vi "Teleop.vi"(10 "Match Info":T1={"Autonomous Elapsed Seconds"=0.0, "TeleOp Elapsed Seconds"=0.0, "Disabled Elapsed Seconds"=0.0, "Visited Autonomous"=FALSE, "Visited TeleOp"=FALSE, "Visited Disabled"=FALSE, "Autonomous Settings"={"Autonomous Style"=enum."Independent", "VI Refnum"=refnum}}, 11 "Call Context":T2) -> ()   [LabVIEW 2014]
doc: "This VI is called for each TeleOp packet received from the DS where the robot is not disabled. It is often used to read from the joysticks and update I/O or to update setpoints for timed control loops. It should complete and return within 20 milliseconds or it may miss DS packets."
uses:
  <vilib>/Rock Robotics/WPI/DriverStation/WPI_DriverStationDerivedRobotMode.ctl
  <vilib>/Rock Robotics/WPI/DriverStation/WPI_DriverStationMatch Info.ctl
  <vilib>/Rock Robotics/WPI/Joystick/WPI_JoystickGetSetRefNum.vi
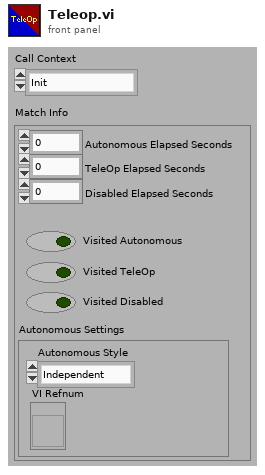
[diagram p1: front panel]
types:
  T1 = typedef "WPI_DriverStationMatch Info.ctl" = cluster{"Autonomous Elapsed Seconds":dbl, "TeleOp Elapsed Seconds":dbl, "Disabled Elapsed Seconds":dbl, "Visited Autonomous":bool, "Visited TeleOp":bool, "Visited Disabled":bool, "Autonomous Settings":cluster{"Autonomous Style":enum16{"Iterative", "Independent"}, "VI Refnum":refnum<vi>}}
  T2 = typedef "WPI_DriverStationDerivedRobotMode.ctl" = enum16{"Init", "Execute", "Stop"}
  T3 = typedef "WPI_SolenoidDevRef.ctl" = cluster{"DevStatus":errorcluster, "Pneumatics Control Module":u8, "Forward Solenoid Channel":T4, "Reverse Solenoid Channel":T4}
  T4 = typedef "WPI_SolenoidChannel.ctl" = enum8{"Solenoid 0", "Solenoid 1", "Solenoid 2", "Solenoid 3", "Solenoid 4", "Solenoid 5", "Solenoid 6", "Solenoid 7", "Invalid"}
  T5 = typedef "WPI_JoystickDevRef.ctl" = cluster{"Device":T6}
  T6 = typedef "WPI_JoystickDeviceEnum.ctl" = enum16{"USB 0", "USB 1", "USB 2", "USB 3", "USB 4", "USB 5"}
  T7 = typedef "WPI_DigitalInputDevRef.ctl" = cluster{"DevStatus":errorcluster, "DIO Channel":T8, "Controller":T9}
  T8 = typedef "FPGA_DIOChannel.ctl" = enum8{"DIO 0", "DIO 1", "DIO 2", "DIO 3", "DIO 4", "DIO 5", "DIO 6", "DIO 7", "DIO 8", "DIO 9", "DIO MXP 0", "DIO MXP 1", "DIO MXP 2", "DIO MXP 3", "DIO MXP 4", "DIO MXP 5", "DIO MXP 6", "DIO MXP 7", "DIO MXP 8", "DIO MXP 9", "DIO MXP 10", "DIO MXP 11", "DIO MXP 12", "DIO MXP 13", "DIO MXP 14", "DIO MXP 15", "Invalid"}
  T9 = typedef "FPGA_TypedefDigitalModule.ctl" = enum16{"Controller 1"}
  T10 = typedef "WPI_AnalogChannelDevRef.ctl" = cluster{"DevStatus":errorcluster, "Controller":T11, "Analog Channel":T12}
  T11 = typedef "FPGA_TypedefAnalogModule.ctl" = enum16{"Controller 1"}
  T12 = typedef "FPGA_AIChannel.ctl" = enum8{"AI 0", "AI 1", "AI 2", "AI 3", "AI MXP 0", "AI MXP 1", "AI MXP 2", "AI MXP 3", "Invalid"}
  T13 = typedef "WPI_MotorControlDeviceRef.ctl" = cluster{"DeviceStatus":errorcluster, "Type":T14, "PWM":cluster{"Controller":T9, "PWM Channel":T15, "DeadBand":T16}, "CAN":cluster{"Device Number":u8, "Control Mode":T17, "Semaphore":T18, "Max Vout":dbl, "TalonSRX Control Mode":T19}, "Invert":bool, "TransformRef":T20, "InvTransformRef":T20}
  T14 = typedef "WPI_MotorControlType.ctl" = enum16{"PWM", "CAN", "CANTalonSRX"}
  T15 = typedef "FPGA_DIOPWMChannel.ctl" = enum8{"PWM 0", "PWM 1", "PWM 2", "PWM 3", "PWM 4", "PWM 5", "PWM 6", "PWM 7", "PWM 8", "PWM 9", "PWM MXP 0", "PWM MXP 1", "PWM MXP 2", "PWM MXP 3", "PWM MXP 4", "PWM MXP 5", "PWM MXP 6", "PWM MXP 7", "PWM MXP 8", "PWM MXP 9", "Invalid"}
  T16 = typedef "WPI_PWMDeadband.ctl" = cluster{"Name":string, "maxPositivePwm":i32, "minPositivePwm":i32, "centerPwm":i32, "maxNegativePwm":i32, "minNegativePwm":i32, "angularRange":u16}
  T17 = typedef "WPI_CANJaguar_ControlMode.ctl" = enum8{"Percent VBus", "Current", "Speed", "Position", "Voltage"}
  T18 = typedef "Semaphore RefNum" = refnum<k1>
  T19 = typedef "WPI_CANTalonSRX_APIControlMode.ctl" = enum8{"Percent VBus", "Speed", "Position", "Slave", "Unchanged / Invalid"}
  T20 = typedef "WPI_PWMTransform_ConPane.ctl" = refnum<vi>
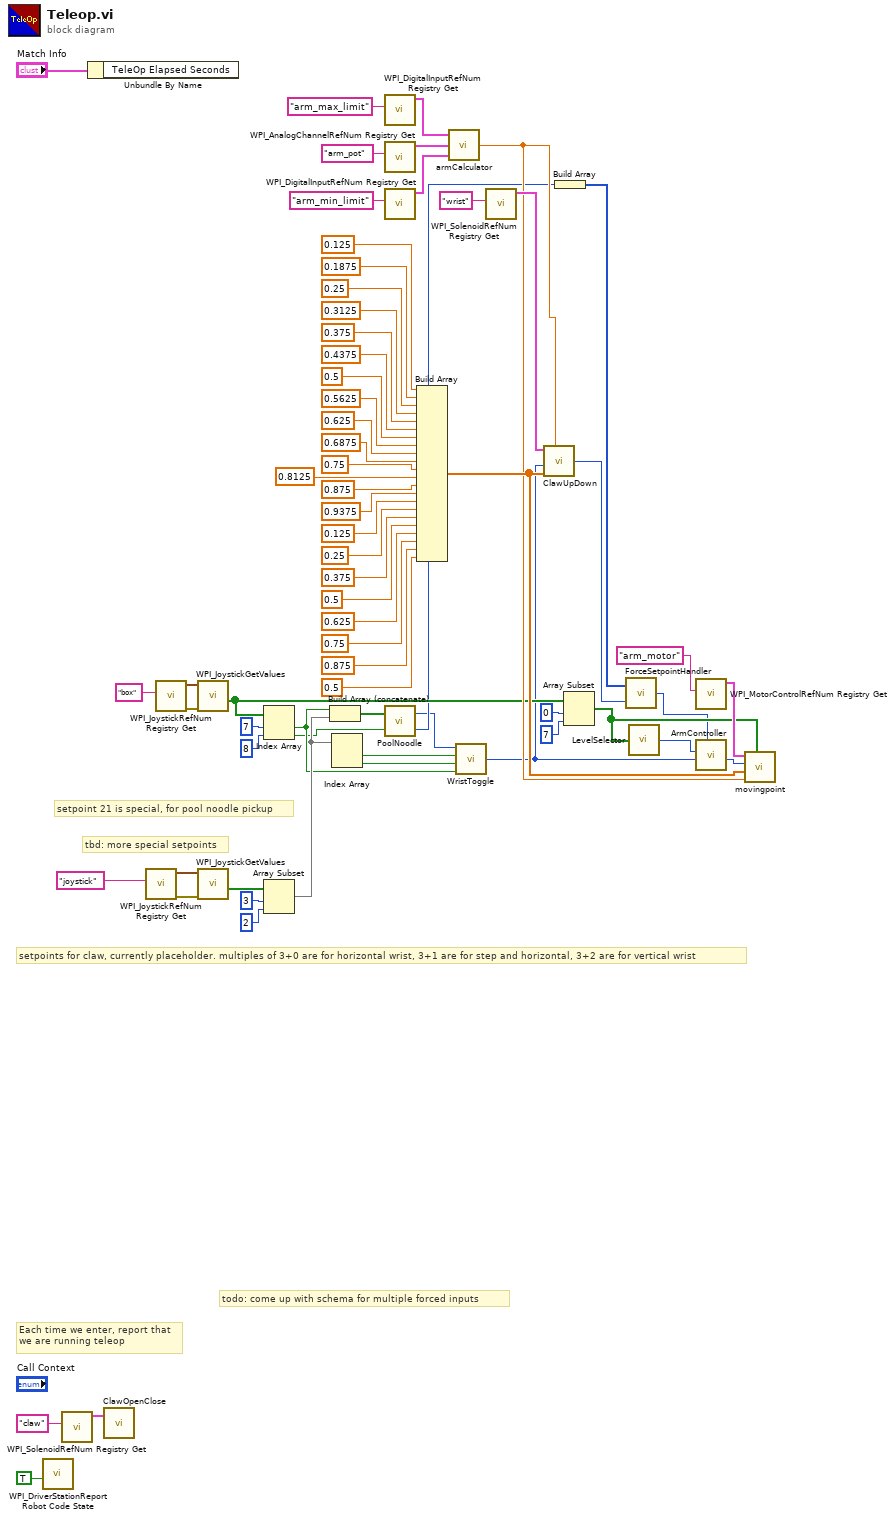
[diagram p0: block diagram]
diagram:
  # "todo: come up with schema for multiple forced inputs"
  # "tbd: more special setpoints"
  # "setpoint 21 is special, for pool noodle pickup"
  # "setpoints for claw, currently placeholder. multiples of 3+0 are for horizontal wrist, 3+1 are for step and horizontal, 3+2 are for vertical wrist"
  # "Each time we enter, report that\nwe are running teleop"
  n1 = call <vilib>:"WPI_DriverStationReport Robot Code State.vi"("TeleOp"=TRUE ("Autonomous")) -> ()  [unwired: 10 in, 1 out]
  n2 = call <vilib>:"WPI_SolenoidRefNum Registry Get.vi"("refnum name"="claw") -> ("SolenoidDevRef"=w58:T3)  [unwired: 9 in, 1 out]
  n3 = Unbundle By Name("Match Info") -> ()  [unwired: 1 out]
  n4 = call "ClawOpenClose.vi"("Claw"=w58) -> ()  [unwired: 2 in]
  n5 = call <vilib>:"WPI_JoystickRefNum Registry Get.vi"("refnum name"="joystick") -> ("error out"=w28:errorcluster, "JoystickDevRef"=w27:T5)  [unwired: 9 in]
  n6 = call <vilib>:"WPI_JoystickRefNum Registry Get.vi"("refnum name"="box") -> ("error out"=w54:errorcluster, "JoystickDevRef"=w53:T5)  [unwired: 9 in]
  n7 = call <vilib>:"WPI_JoystickGetValues.vi"("error in (no error)"=w54, "JoystickDevRef"=w53) -> ("Buttons"=w26:bool[])  [unwired: 5 in, 4 out]
  n8 = call <vilib>:"WPI_JoystickGetValues.vi"("error in (no error)"=w28, "JoystickDevRef"=w27) -> ("Buttons"=w24:bool[])  [unwired: 5 in, 4 out]
  n9 = Index Array(array=w26, index #1=7 ("index"), index #2=8 ("index")) -> (element #1=w6:bool, element #2=w3:bool)
  n10 = Array Subset(array=w24, index=3, length=2) -> (w21:bool[])
  n11 = Build Array (concatenate)(w6, w21) -> (w2:bool[])
  n12 = Index Array(array=w21) -> (element #1=w8:bool, element #2=w7:bool)  [unwired: 2 in]
  n13 = call <vilib>:"WPI_DigitalInputRefNum Registry Get.vi"("refnum name"="arm_max_limit") -> ("DigitalInputDevRef"=w63:T7)  [unwired: 9 in, 1 out]
  n14 = call <vilib>:"WPI_AnalogChannelRefNum Registry Get.vi"("refnum name"="arm_pot") -> ("AIDeviceRef"=w61:T10)  [unwired: 9 in, 1 out]
  n15 = call <vilib>:"WPI_DigitalInputRefNum Registry Get.vi"("refnum name"="arm_min_limit") -> ("DigitalInputDevRef"=w62:T7)  [unwired: 9 in, 1 out]
  n16 = call "PoolNoodle.vi"("Input"=w3, "State Buttons"=w2) -> ("Force Pool Noodle"=w5:i32, "Force State"=w4:i32)
  n17 = Build Array(0.125, 0.1875 ("element"), 0.25 ("element"), 0.3125 ("element"), 0.375 ("element"), 0.4375 ("element"), 0.5 ("element"), 0.5625 ("element"), 0.625 ("element"), 0.6875 ("element"), 0.75 ("element"), 0.8125 ("element"), 0.875 ("element"), 0.9375 ("element"), 0.125 ("element"), 0.25 ("element"), 0.375 ("element"), 0.5 ("element"), 0.625 ("element"), 0.75 ("element"), 0.875 ("element"), 0.5 ("element")) -> (w36:dbl[])
  n18 = call "armCalculator.vi"("Min Limit Switch"=w62, "AIDeviceRef"=w61, "Max Limit Switch"=w63) -> ("Scaled Pot Val"=w35:dbl)
  n19 = call "WristToggle.vi"("Step Control"=w6, "Vertical Control"=w7, "Horizontal Control"=w8, "Force State"=w4) -> ("State"=w1:i32)
  n20 = call <vilib>:"WPI_SolenoidRefNum Registry Get.vi"("refnum name"="wrist") -> ("SolenoidDevRef"=w37:T3)  [unwired: 9 in, 1 out]
  n21 = call "ClawUpDown.vi"("Wrist"=w37, "Scaled Pot"=w35, "State"=w1, "Setpoints"=w36) -> ("SetpointOut"=w10:i32)  [unwired: 4 in]
  n22 = Build Array(w5) -> (w9:i32[])
  n23 = Array Subset(array=w26, index=0, length=7) -> (w30:bool[])
  n24 = call "ForceSetpointHandler.vi"("Wrist Force"=w10, "Force Setpoints"=w9) -> ("Force Setpoint"=w11:i32)
  n25 = call "LevelSelector.vi"("Buttons"=w30) -> ("Level"=w33:i32)
  n26 = call <vilib>:"WPI_MotorControlRefNum Registry Get.vi"("refnum name"="arm_motor") -> ("MotorControlDevRef"=w38:T13)  [unwired: 9 in, 1 out]
  n27 = call "ArmController.vi"("Force Value"=w11, "State"=w1, "Level"=w33) -> ("Setpoint"=w34:i32)  [unwired: 8 in]
  n28 = call "movingpoint.vi"("Buttons"=w30, "Pot Scaled Value"=w35, "Setpoints"=w36, "Setpoint Index"=w34, "MotorControlDevRef"=w38) -> ()  [unwired: 6 in, 1 out]
